vi "Create App.vi"(9 "Alias":string, 10 "Nest Actor":refnum<class "LVCAM.lvclass">) -> (0 "error out":errorcluster)   [LabVIEW 2021, in "LVCAM.lvlib" / "Self Actor.lvclass"]
uses:
  Self Actor.lvclass
  LVCAM/LVCAM.lvclass
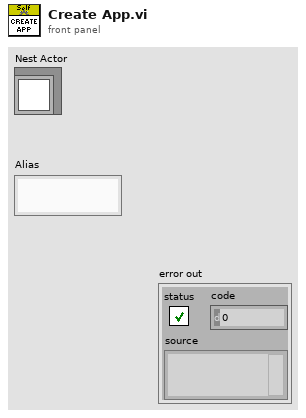
[diagram p1: front panel]
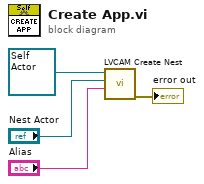
[diagram p0: block diagram]
diagram:
  n1 = call-dynamic "LVCAM Create Nest.vi"("Alias"="Alias", "Nest Actor"="Nest Actor", "Self Actor in"=refnum<class "Self Actor.lvclass"> refnum) -> ("error out"=→"error out":errorcluster)  [unwired: 7 in, 1 out]
